vi "_Buffer_To_ElementAtIndex.vi"(10 "index (-1: last)":i32=-1, 11 "Buffer":refnum<class "VariantBuffer.lvclass">) -> (1 "found":bool, 3 "element":variant)   [LabVIEW 2013, in "VariantBuffer.lvclass"]
uses:
  VariantBuffer.lvclass
  VariantBuffer.lvclass/VariantBuffer.ctl
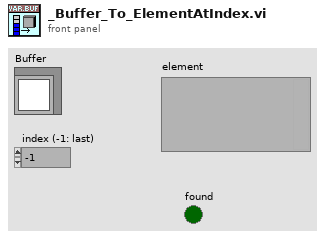
[diagram p1: front panel]
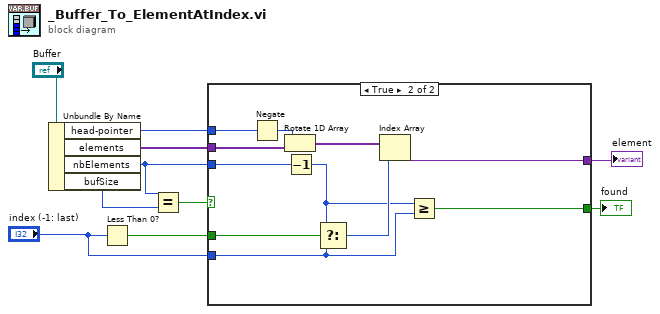
[diagram p0: block diagram]
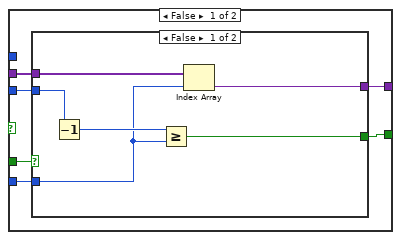
[diagram p2: hidden frame]
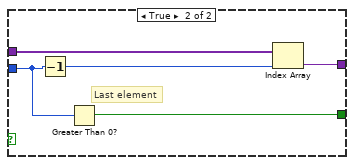
[diagram p3: hidden frame]
diagram:
  n1 = Unbundle By Name("Buffer") -> ("head-pointer"=w8:i32, "elements"=w6:variant[], "nbElements"=w10:i32, "bufSize"=w9:i32)
  n2 = Less Than 0?(x="index (-1: last)") -> (x < 0?=w3:bool)
  n3 = Equal?(x=w10, y=w9) -> (x = y?=w5:bool)
  n4 = case shown="True" w5 {
    tunnel: w6 -> [w15 w38]
    tunnel: w8 -> [_ w36]
    tunnel: w10 -> [w16 w33]
    tunnel: [w14 w28] -> w4
    tunnel: w3 -> [w13 w34]
    tunnel: "index (-1: last)" -> [w12 w30]
    tunnel: [w11 w29] -> w1
    frame False {
      n5 = case shown="False" w13 {
        tunnel: w16 -> [w20 w24]
        tunnel: w15 -> [w22 w27]
        tunnel: [w21 w26] -> w14
        tunnel: w12 -> [w18 _]
        tunnel: [w17 w23] -> w11
        frame False {
          n6 = Decrement(x=w20) -> (x-1=w19:i32)
          n7 = Greater Or Equal?(x=w19, y=w18) -> (x >= y?=w17:bool)
          n8 = Index Array(array=w22, index=w18) -> (element=w21:variant)
        }
        frame True {
          # "Last element"
          n9 = Decrement(x=w24) -> (x-1=w25:i32)
          n10 = Greater Than 0?(x=w24) -> (x > 0?=w23:bool)
          n11 = Index Array(array=w27, index=w25) -> (element=w26:variant)
        }
      }
    }
    frame True {
      n12 = Negate(x=w36) -> (-x=w37:i32)
      n13 = Rotate 1D Array(1:w38, 2:w37) -> (0:w35:variant[])
      n14 = Decrement(x=w33) -> (x-1=w31:i32)
      n15 = Select(t=w31, s=w34, f=w30) -> (s? t:f=w32:i32)
      n16 = Index Array(array=w35, index=w32) -> (element=w28:variant)
      n17 = Greater Or Equal?(x=w31, y=w30) -> (x >= y?=w29:bool)
    }
  }
  "element" <- w4
  "found" <- w1
